vi "PurgeTime.vi"(10 "Cluster":T1={"PWM"=0, "PurgeStart"=TRUE, "DKG"=TRUE, "Purge Time"=0}) -> (2 "Purge Time":dbl)   [LabVIEW 2017]
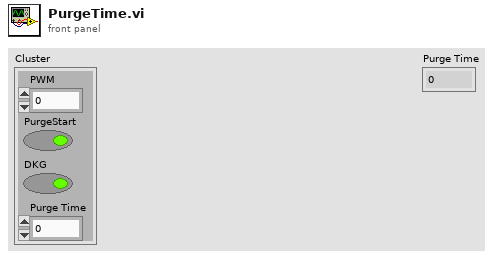
[diagram p1: front panel]
types:
  T1 = cluster{"PWM":i32, "PurgeStart":bool, "DKG":bool, "Purge Time":i32}
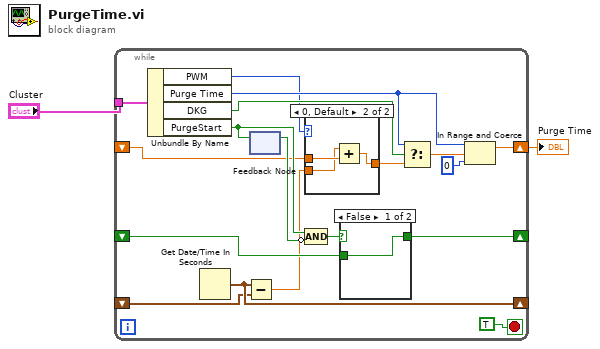
[diagram p0: block diagram]
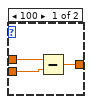
[diagram p2: hidden frame]
diagram:
  n1 = while {
    tunnel: "Cluster" -> [w19]
    shift-right: [w14] -> w1
    shift-left: _ -> [w5]
    shift-right: [w10] -> _
    shift-left: _ -> [w9]
    shift-right: [w8] -> _
    shift-left: _ -> [w7]
    stop <- TRUE stop-if-true
    n2 = Unbundle By Name(w19) -> ("PWM"=w6:i32, "Purge Time"=w13:i32, "DKG"=w16:bool, "PurgeStart"=w18:bool)
    n3 = Get Date/Time In Seconds() -> (seconds since 1Jan1904=w8:timestamp)
    n4 = Subtract(x=w8, y=w7) -> (x-y=w4:dbl)
    n5 = feedback #1() -> (w17:bool)  [unwired: 1 in]
    n6 = feedback-in #1(w18) -> ()
    n7 = case shown="0, Default" w6 {
      tunnel: w5 -> [w23 w26]
      tunnel: w4 -> [w22 w25]
      tunnel: [w21 w24] -> w3
      frame 100 {
        n8 = Subtract(x=w23, y=w22) -> (x-y=w21:dbl)
      }
      frame 0, Default {
        n9 = Add(x=w25, y=w26) -> (x+y=w24:dbl)
      }
    }
    n10 = Compound Arithmetic op=AND(w18, invert w17) -> (w11:bool)
    n11 = case shown="False" w11 {
      selector: w11 -> [_ w28]
      tunnel: [w27 w28] -> w10
      tunnel: w9 -> [w27 _]
      frame False {
      }
      frame True {
      }
    }
    n12 = Select(t=w13, s=w16, f=w3) -> (s? t:f=w15:dbl)
    n13 = In Range and Coerce(upper limit=w13, x=w15, lower limit=0) -> (coerced(x)=w14:dbl)  [unwired: 1 out]
  }
  "Purge Time" <- w1
